vi "Test Vector.vi"(8 "error in (no error)":errorcluster, 11 "Test Vector Demo In":refnum<class "Test Vector Demo.lvclass">) -> (0 "error out":errorcluster, 3 "Test Vector Demo Out":refnum<class "Test Vector Demo.lvclass">)   [LabVIEW 2020, in "Test Vector Demo.lvclass"]
doc: "This test method executes the test vector on the VI under test, which all are configured using the methods available. A vector consists of multiple components where each component is a single test. A component is defined by setting control input values and expected results for the component. When the test case is run, controls are reinitialized to default values, the configured inputs are set, the VI is run and the outputs are compared against the expected results."
uses:
  Test Vector Demo.lvclass
  C:/Users/anton/Documents/GitHub/LUnit/source/Framework/Test Vector/LUnit Test Vector.lvclass
  Framework/Test Vector/LUnit Test Vector.lvclass/LUnit Test Vector.ctl
  Framework/Test Vector/LUnit Test Vector.lvclass
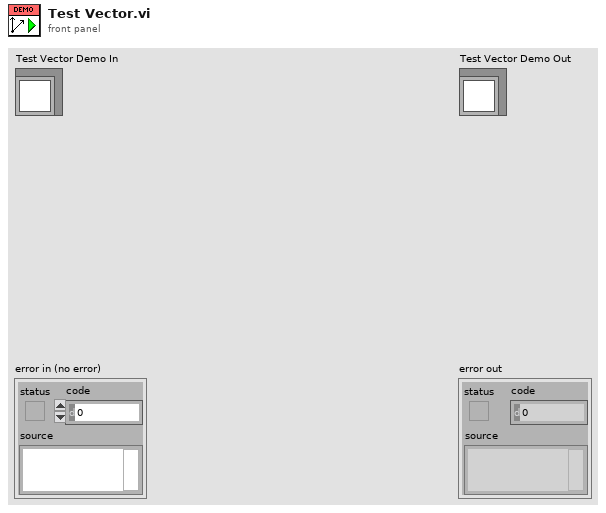
[diagram p1: front panel]
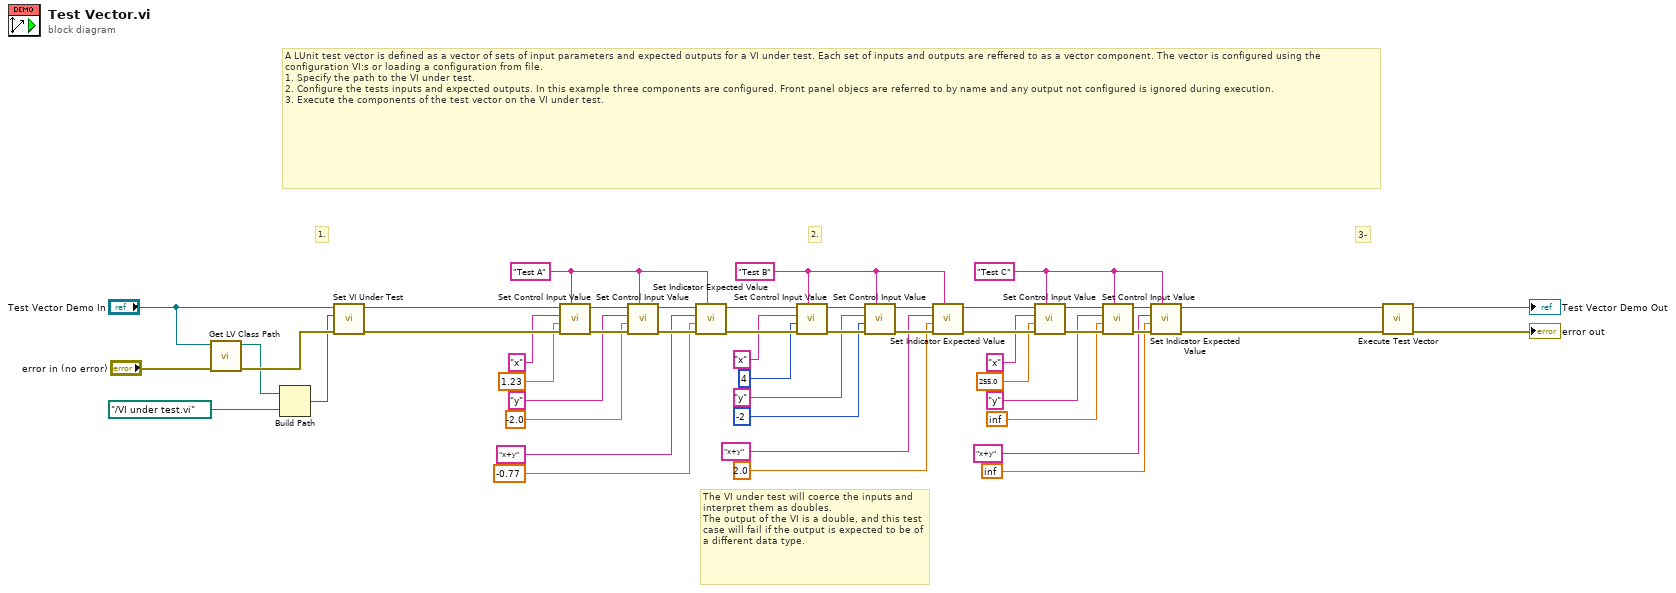
[diagram p0: block diagram]
diagram:
  w1 = "Test C" ("Vector Component")
  w22 = "Test B" ("Vector Component")
  w31 = "Test A" ("Vector Component")
  # "3-"
  # "2."
  # "1."
  # "A LUnit test vector is defined as a vector of sets of input parameters and expected outputs for a VI under test. Each set of inputs and outputs are reffered to as a vector component. The vector is configured using the configuration VI:s or loading a configuration from file.\n1. Specify the path to the VI under test.\n2. Configure the tests inputs and expected outputs. In this example three components are configured. Front panel objecs are referred to by name and any output not configured is ignored during execution.\n3. Execute the components of the test vector on the VI under test."
  # "The VI under test will coerce the inputs and interpret them as doubles. \nThe output of the VI is a double, and this test case will fail if the output is expected to be of a different data type."
  n1 = call <vilib>:"Get LV Class Path.vi"("error in (no error)"="error in (no error)", "object"="Test Vector Demo In") -> ("error out"=w11:errorcluster, "class path"=w10:path)  [unwired: 8 in]
  n2 = Build Path(base path=w10, name or relative path=path "../VI under test.vi" ("VI Under Test Path")) -> (appended path=w8:path)
  n3 = call "Set VI Under Test.vi"("error in (no error)"=w11, "VI Under Test Path"=w8, "LUnit Test Vector In"="Test Vector Demo In") -> ("error out"=w46:errorcluster, "LUnit Test Vector Out"=w47:refnum<class "Test Vector Demo.lvclass">)  [unwired: 7 in]
  n4 = call "Set Control Input Value.vi"("Vector Component"=w31, "error in (no error)"=w46, "Data"=1.23, "Control Name"="x", "LUnit Test Vector In"=w47) -> ("error out"=w44:errorcluster, "LUnit Test Vector Out"=w45:refnum<class "Test Vector Demo.lvclass">)  [unwired: 5 in]
  n5 = call "Set Control Input Value.vi"("Vector Component"=w31, "error in (no error)"=w44, "Data"=-2.0, "Control Name"="y", "LUnit Test Vector In"=w45) -> ("error out"=w42:errorcluster, "LUnit Test Vector Out"=w43:refnum<class "Test Vector Demo.lvclass">)  [unwired: 5 in]
  n6 = call "Set Indicator Expected Value.vi"("Vector Component"=w31, "error in (no error)"=w42, "Data"=-0.77, "Control Name"="x+y", "LUnit Test Vector In"=w43) -> ("error out"=w40:errorcluster, "LUnit Test Vector Out"=w41:refnum<class "Test Vector Demo.lvclass">)  [unwired: 5 in]
  n7 = call "Set Control Input Value.vi"("Vector Component"=w22, "error in (no error)"=w40, "Data"=4, "Control Name"="x", "LUnit Test Vector In"=w41) -> ("error out"=w38:errorcluster, "LUnit Test Vector Out"=w39:refnum<class "Test Vector Demo.lvclass">)  [unwired: 5 in]
  n8 = call "Set Control Input Value.vi"("Vector Component"=w22, "error in (no error)"=w38, "Data"=-2, "Control Name"="y", "LUnit Test Vector In"=w39) -> ("error out"=w36:errorcluster, "LUnit Test Vector Out"=w37:refnum<class "Test Vector Demo.lvclass">)  [unwired: 5 in]
  n9 = call "Set Indicator Expected Value.vi"("Vector Component"=w22, "error in (no error)"=w36, "Data"=2.0, "Control Name"="x+y", "LUnit Test Vector In"=w37) -> ("error out"=w34:errorcluster, "LUnit Test Vector Out"=w35:refnum<class "Test Vector Demo.lvclass">)  [unwired: 5 in]
  n10 = call "Set Control Input Value.vi"("Vector Component"=w1, "error in (no error)"=w34, "Data"=255.0, "Control Name"="x", "LUnit Test Vector In"=w35) -> ("error out"=w32:errorcluster, "LUnit Test Vector Out"=w33:refnum<class "Test Vector Demo.lvclass">)  [unwired: 5 in]
  n11 = call "Set Control Input Value.vi"("Vector Component"=w1, "error in (no error)"=w32, "Data"=inf, "Control Name"="y", "LUnit Test Vector In"=w33) -> ("error out"=w5:errorcluster, "LUnit Test Vector Out"=w7:refnum<class "Test Vector Demo.lvclass">)  [unwired: 5 in]
  n12 = call "Set Indicator Expected Value.vi"("Vector Component"=w1, "error in (no error)"=w5, "Data"=inf, "Control Name"="x+y", "LUnit Test Vector In"=w7) -> ("error out"=w4:errorcluster, "LUnit Test Vector Out"=w6:refnum<class "Test Vector Demo.lvclass">)  [unwired: 5 in]
  n13 = call "Execute Test Vector.vi"("error in (no error)"=w4, "LUnit Test Vector in"=w6) -> ("error out"=→"error out":errorcluster, "LUnit Test Vector out"=→"Test Vector Demo Out":refnum<class "Test Vector Demo.lvclass">)  [unwired: 8 in]
